vi "Advance_Gauge_TL_SubVi.vi"(11 "Knob in":refnum<vi>) -> (3 "Gauge":dbl(knob) scale=0.0..100.0)   [LabVIEW 2014]
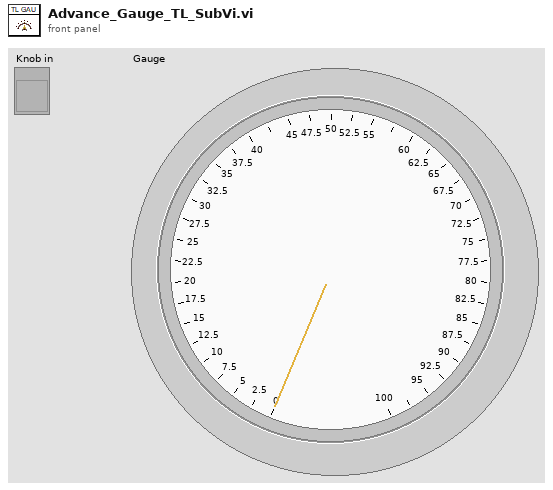
[diagram p1: front panel]
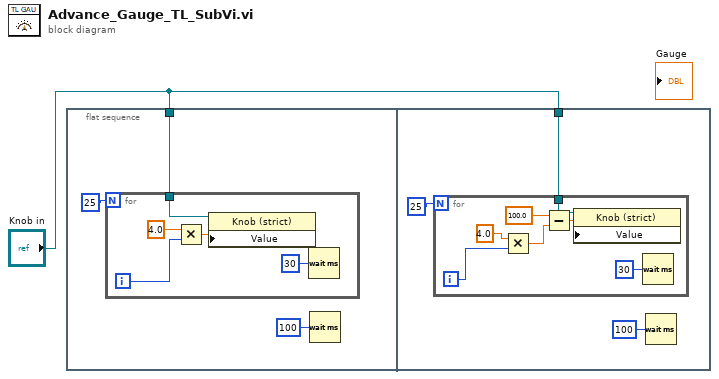
[diagram p0: block diagram]
diagram:
  n1 = flat-sequence {
    tunnel: "Knob in" -> [w2]
    tunnel: "Knob in" -> [w10]
    frame #0 {
      n2 = for {
        N: 25 -> [_]
        tunnel: w2 -> [w6]
        i -> [w5]
        n3 = Multiply(x=4.0, y=w5) -> (x*y=w7:dbl)
        n4 = property class="Knob (strict)"(reference=w6, "Value"=w7) -> ()  [unwired: 1 in, 2 out]
        n5 = Wait (ms)(milliseconds to wait=u32 30) -> ()  [unwired: 1 out]
      }
      n6 = Wait (ms)(milliseconds to wait=u32 100) -> ()  [unwired: 1 out]
    }
    frame #1 {
      n7 = for {
        N: 25 -> [_]
        tunnel: w10 -> [w13]
        i -> [w15]
        n8 = Multiply(x=4.0, y=w15) -> (x*y=w16:dbl)
        n9 = Subtract(x=100.0, y=w16) -> (x-y=w14:dbl)
        n10 = property class="Knob (strict)"(reference=w13, "Value"=w14) -> ()  [unwired: 1 in, 2 out]
        n11 = Wait (ms)(milliseconds to wait=u32 30) -> ()  [unwired: 1 out]
      }
      n12 = Wait (ms)(milliseconds to wait=u32 100) -> ()  [unwired: 1 out]
    }
  }
